vi "PCSMain.destructor.vi"(0 "i ref in":refnum<vi>, 5 "error in":errorcluster) -> (19 "error out":errorcluster)   [LabVIEW 2014, in "PCSMain.lvlib"]
doc: "This is the destructor of a class.\n\nLicense Agreement for this software:\n\nCopyright (C)\nGesellschaft für Schwerionenforschung, GSI\nPlanckstr. 1\n64291 Darmstadt\nGermany\n\nContact: D.Beck@gsi.de \n\nThis program is free software; you can redistribute it and/or modify it under the terms of the \nGNU General Public License as published by the Free Software Foundation; either version 2 of \nthe license, or (at your option) any later version.\n\nThis program is distributed in the hope that it will be useful, but WITHOUT ANY WARRANTY; \nwithout even the implied warranty of MERCHANTABILITY or FITNESS FOR A PARTICULAR PURPOSE. See the GNU General License for more details (http://www.gnu.org).\n\nGesellschaft für Schwerionenforschung, GSI\nPlanckstr. 1, 64291 Darmstadt, Germany\nFor all questions and ideas contact: M.Richter@gsi.de, H.Brand@gsi.de or D.Beck@gsi.de.\nLast update: 16-JUN-2004"
uses:
  PCSMain.lvlib
  CSCore/BaseGUI/BaseGUI.lvlib
  PH_Common/PH_Common.lvlib
  CSCore/CSObj/CSObj.lvlib
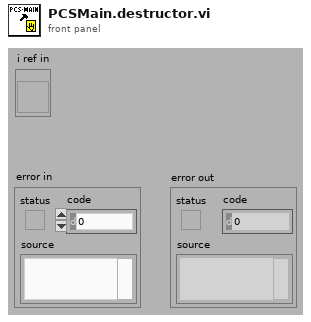
[diagram p1: front panel]
types:
  T1 = enum16{"SetAttribute", "GetAttribute", "CreateAttribute", "DestroyAttribute", "DestroyAllAtributes"}
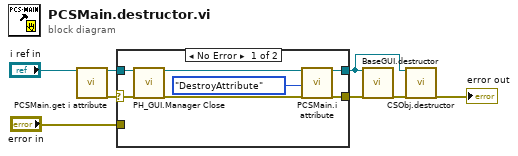
[diagram p0: block diagram]
diagram:
  n1 = call "PCSMain.get i attribute.vi"("i ref in"="i ref in") -> ("i ref out"=w3:refnum<vi>, "error out"=w5:errorcluster)  [unwired: 16 in, 1 out]
  n2 = case shown="No Error" w5 {
    selector: w5 -> [w13 _]
    tunnel: [w9 w16] -> w7
    tunnel: w3 -> [w14 w17]
    tunnel: [w11 w17] -> w1
    tunnel: "error in" -> [_ w16]
    frame No Error {
      n3 = call "PH_GUI.Manager Close.vi"("i ref in"=w14, "error in"=w13) -> ("i ref out"=w12:refnum<vi>, "error out"=w10:errorcluster)  [unwired: 16 in]
      n4 = call "PCSMain.i attribute.vi"("VI Refnum"=w12, "Action"=T1."DestroyAttribute", "error in (no error)"=w10) -> ("VI Refnum out"=w11:refnum<vi>, "error out"=w9:errorcluster)  [unwired: 14 in, 1 out]
    }
    frame Error {
    }
  }
  n5 = call "BaseGUI.destructor.vi"("i ref in"=w1, "error in (no error)"=w7) -> ("error out"=w8:errorcluster)  [unwired: 17 in]
  n6 = call "CSObj.destructor.vi"("i ref in"=w1, "error in (no error)"=w8) -> ("error out"=→"error out":errorcluster)  [unwired: 17 in]
